vi "Untitled 5 (SubVI)1111.vi"(11 "Tx":dbl) -> (3 "Numeric":dbl)   [LabVIEW 2020]
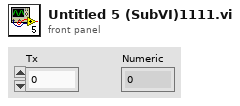
[diagram p1: front panel]
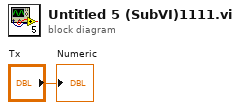
[diagram p0: block diagram]
diagram:
  "Numeric" <- "Tx"
